vi "ConfigAppearance.vi"(8 "error in (no error)":errorcluster, 10 "Column Appearance":T1={"Column Name"="", "Width"=30, "Bkgd"=[16448250], "Text"=[0]}, 11 "Column in":refnum<class "Column.lvclass">) -> (0 "error out":errorcluster, 3 "Column out":refnum<class "Column.lvclass">)   [LabVIEW 2013, in "Column.lvclass"]
uses:
  Column.lvclass
  TypeDefs/ColumnAppearCluster.ctl
  Column.lvclass/Column.ctl
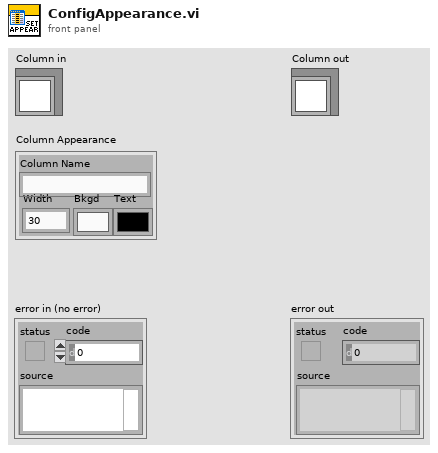
[diagram p1: front panel]
types:
  T1 = typedef "ColumnAppearCluster.ctl" = cluster{"Column Name":string, "Width":u32, "Bkgd":u32[], "Text":u32[]}
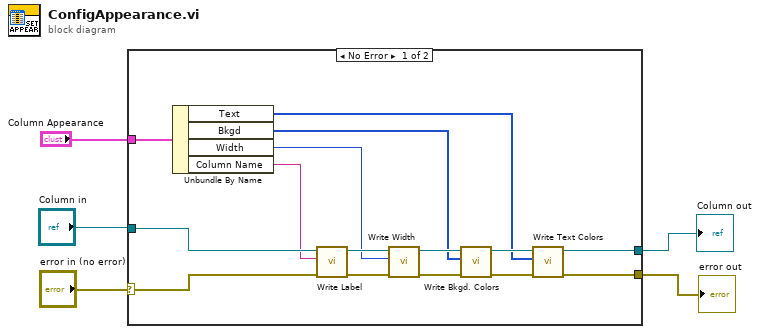
[diagram p0: block diagram]
diagram:
  n1 = case shown="No Error" "error in (no error)" {
    selector: "error in (no error)" -> [w13 w22]
    tunnel: [w6 w22] -> w2
    tunnel: [w7 w21] -> w1
    tunnel: "Column in" -> [w17 w21]
    tunnel: "Column Appearance" -> [w12 _]
    frame No Error {
      n2 = Unbundle By Name(w12) -> ("Text"=w8:u32[], "Bkgd"=w9:u32[], "Width"=w10:u32, "Column Name"=w11:string)
      n3 = call "Write Label.vi"("error in (no error)"=w13, "Label"=w11, "Column in"=w17) -> ("error out"=w16:errorcluster, "Column out"=w20:refnum<class "Column.lvclass">)  [unwired: 7 in]
      n4 = call "Write Width.vi"("error in (no error)"=w16, "Width"=w10, "Column in"=w20) -> ("error out"=w15:errorcluster, "Column out"=w19:refnum<class "Column.lvclass">)  [unwired: 7 in]
      n5 = call "Write Bkgd. Colors.vi"("error in (no error)"=w15, "Bkgd. Colors"=w9, "Column in"=w19) -> ("error out"=w14:errorcluster, "Column out"=w18:refnum<class "Column.lvclass">)  [unwired: 7 in]
      n6 = call "Write Text Colors.vi"("error in (no error)"=w14, "Text Colors"=w8, "Column in"=w18) -> ("error out"=w6:errorcluster, "Column out"=w7:refnum<class "Column.lvclass">)  [unwired: 7 in]
    }
    frame Error {
    }
  }
  "error out" <- w2
  "Column out" <- w1
